vi "Gh为空报警.vi"(10 "油动机实验报告":T1, 11 "保存数据输入":bool) -> (0 "保存2":bool, 3 "flag":bool)   [LabVIEW 2013]
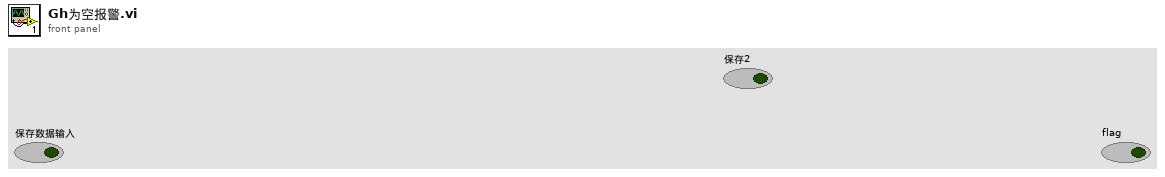
[diagram p1: front panel]
types:
  T1 = cluster{"油动机试验报告名称":string, "供应商1":string, "合同号1":string, "数量1":string, "用户1":string, "订货号1":string, "订货日期1":string, "项目名称1":string, "油动机图号2.1":string, "油动机系列号2.1":string, "阀门行程Vh":string, "试验介质及油质2.2":string, "超行程Oh1":string, "超行程Oh2":string, "粘度2.2":string, "油温2.2":string, "系统压力2.2":string, "油动机型号2.3":string, "运行方式2.3":string, "范围2.3":string, "安装方式2.3":string, "活塞直径D":string, "活塞杆直径d":string, "工作行程Vh2.3":string, "活塞杆引导2.3":string, "油动机型式2.3":string, "连接块2.3":string, "逻辑元件尺寸2.3":string, "杆结构2.3":string, "活塞杆端2.3":string, "缓冲2.3":string, "密封系统2.3":string, "位移传感器2.3":string, "位移传感器量程TS":string, "输出信号":string, "外形尺寸_2.4.1":string, "泄漏试验与否_2.4.1":string, "功能试验与否_2.4.1":string, "最小电压试验与否_2.4.1":string, "压力试验与否_2.4.1":string, "要求起始位2.4.2":string, "实际起始位":string, "要求总行程Gh2.4.2":string, "理论摩擦力F2.4.3":string, "要求灵敏度2.4.2":string, "理论F12.4.3":string, "要求终端位2.4.2":string, "要求阀门零位2.4.2":string, "理论F22.4.3":string, "实际阀门零位V1":string, "实际终端位V2":string, "实际灵敏度SEN":string, "实际总行程Gh":string, "实测F1":string, "实测F2":string, "实测F":string, "油动机在BP位_测量_X":string, "油动机在BP位_测量_Y":string, "油动机在BP位_测量_Z":string, "要求开关延时_开启2.4.5":string, "实际OP":string, "要求开关延时_关闭2.4.5":string, "实际CL":string, "要求开关延时_归零2.4.5":string, "实际DFT":string, "泄油节油孔1_BI1_2.4.5":string, "泄油节油孔2_BI2_2.4.5":string, "要求延迟时间tv_2.4.5":string, "要求总关闭时间ts_2.4.5":string, "要求_终端速度_2.4.6":string, "要求_长度_2.4.6":string, "要求_放油孔直径_2.4.6":string, "要求_节流孔直径_2.4.6":string, "延迟时间L1L2":string, "延迟时间L1":string, "延迟时间L2":string, "总关闭时间L1L2":string, "总关闭时间L1":string, "总关闭时间L2":string, "实际_节流孔直径_2.4.6":string, "缓冲时间td":string, "实际终端速度":string, "实际_长度_2.4.6":string, "实际_放油孔直径_2.4.6":string, "要求_缓冲时间_2.4.6":string, "控制器放大倍数_2.4.7":string, "伸出实测_控制器放大倍数_2.4.7":string, "缩入实测_控制器放大倍数_2.4.7":string, "要求_全程时间_2.4.7":string, "要求_过调时间_2.4.7":string, "要求_过调量_2.4.7":string, "伸出实测_全程时间":string, "伸出实测_过调量":string, "伸出实测_过调时间":string, "缩入实测_全程时间":string, "缩入实测_过调量":string, "缩入实测_过调时间":string, "堵塞指示_2.4.8":string, "法兰_2.4.8 ":string, "铭牌_2.4.8 ":string, "机械行程指示_2.4.8 ":string, "低漆_2.5":string, "面漆_2.5":string, "名称_2.6":string, "启动阀_供应商_2.6":string, "启动阀_型号_2.6":string, "启动阀_系列号_2.6":string, "启动阀_编号_2.6":string, "位移变送器_供应商_2.6":string, "位移变送器_型号_2.6":string, "位移变送器_系列号_2.6":string, "位移变送器_编号_2.6":string, "主门至全开位_2.7":string, "调门至V1位_2.7":string}
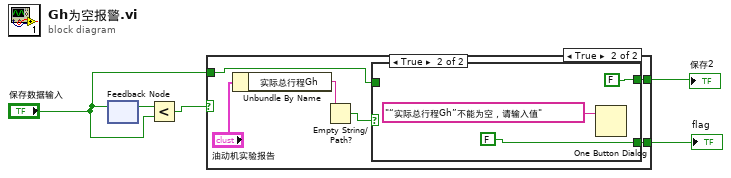
[diagram p0: block diagram]
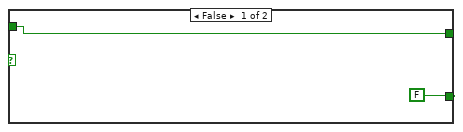
[diagram p2: hidden frame]
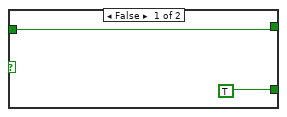
[diagram p3: hidden frame]
diagram:
  n1 = feedback #1() -> (w3:bool)  [unwired: 1 in]
  n2 = feedback-in #1("保存数据输入") -> ()
  n3 = Less?(x=w3, y="保存数据输入") -> (x < y?=w4:bool)
  n4 = case shown="True" w4 {
    tunnel: [FALSE ("保存数据") w10] -> w5
    tunnel: [w6 w9] -> w2
    tunnel: "保存数据输入" -> [w6 w8]
    frame False {
    }
    frame True {
      n5 = Unbundle By Name("油动机实验报告") -> ("实际总行程Gh"=w12:string)
      n6 = Empty String/Path?(string/path=w12) -> (empty?=w11:bool)
      n7 = case shown="True" w11 {
        tunnel: [TRUE ("保存数据") FALSE ("保存数据")] -> w10
        tunnel: [w14 FALSE ("保存数据")] -> w9
        tunnel: w8 -> [w14 _]
        frame False {
        }
        frame True {
          n8 = One Button Dialog(message="“实际总行程Gh”不能为空，请输入值" ("消息")) -> ()  [unwired: 1 in, 1 out]
        }
      }
    }
  }
  "flag" <- w5
  "保存2" <- w2
